vi "ENA_Wait For Operation Complete.vi"(8 "error in (no error)":errorcluster, 11 "VISA resource name":refnum<visa-resource-name>) -> (0 "error out":errorcluster, 3 "VISA resource name out":refnum<visa-resource-name>)   [LabVIEW 2013]
doc: "Waits for the operation to complete."
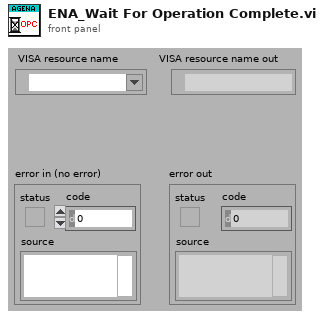
[diagram p1: front panel]
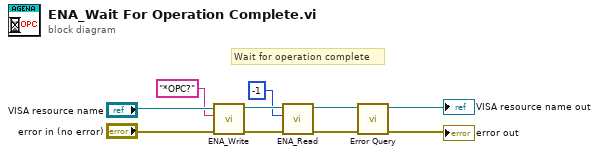
[diagram p0: block diagram]
diagram:
  # "Wait for operation complete"
  n1 = call "ENA_Write.vi"("error in (no error)"="error in (no error)", "String ()"="*OPC?" ("write buffer"), "VISA resource name"="VISA resource name") -> ("error out"=w6:errorcluster, "VISA resource name out"=w7:refnum<visa-resource-name>)  [unwired: 6 in, 1 out]
  n2 = call "ENA_Read.vi"("error in (no error)"=w6, "Number Of Bytes"=-1 ("byte count"), "VISA resource name"=w7) -> ("error out"=w3:errorcluster, "VISA resource name out"=w4:refnum<visa-resource-name>)  [unwired: 5 in, 2 out]
  n3 = call "Error Query.vi"("error in (no error)"=w3, "VISA resource name"=w4) -> ("error out"=→"error out":errorcluster, "VISA resource name out"=→"VISA resource name out":refnum<visa-resource-name>)  [unwired: 6 in, 2 out]
